vi "Codec_defaultJSON.vi"(8 "error in (no error)":errorcluster, 11 "SecureMqttCodec in":refnum<class "SecureMqttCodec.lvclass">) -> (0 "error out":errorcluster, 3 "SecureMqttCodec out":refnum<class "SecureMqttCodec.lvclass">)   [LabVIEW 2020, in "SecureMqttCodec.lvclass"]
uses:
  SecureMqttCodec.lvclass
  SecureMqttCodec.lvclass/SecureMqttCodec.ctl
  <vilib>/addons/JSON API/JSON Value/Set from JSON string.vi
  <vilib>/LabVIEW Open Source Project/Epoch Date & Time/epoch.UNIX/Epoch.UNIX.lvclass
  C:/Program Files/National Instruments/LabVIEW 2020/vi.lib/LabVIEW Open Source Project/Epoch Date & Time/epoch/Epoch.lvclass
  <vilib>/addons/JSON API/JSON Scalar/JSON Scalar.lvclass
  C:/Program Files/National Instruments/LabVIEW 2020/vi.lib/addons/JSON API/JSON Value/JSON Value.lvclass
  <vilib>/LabVIEW Open Source Project/Epoch Date & Time/Get Epoch Time.vi
  <vilib>/addons/JSON API/JSON Scalar/Set I64.vi
  <vilib>/addons/JSON API/JSON Scalar/Set String.vi
  <vilib>/addons/JSON API/JSON Value/JSON Value.lvclass
  <vilib>/addons/JSON API/Get Polymorphic/JSON GetSet.lvlib
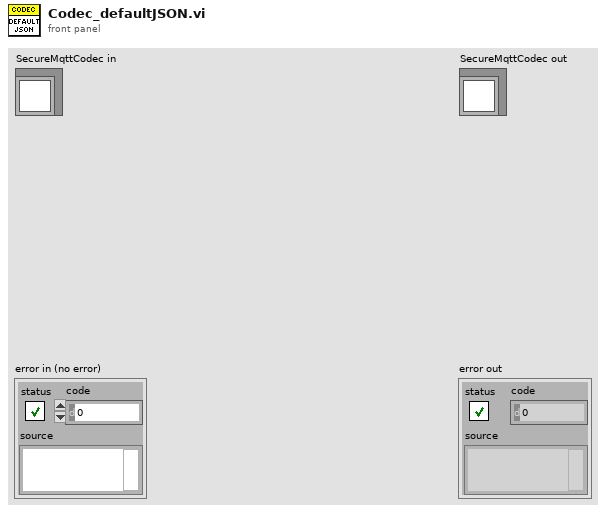
[diagram p1: front panel]
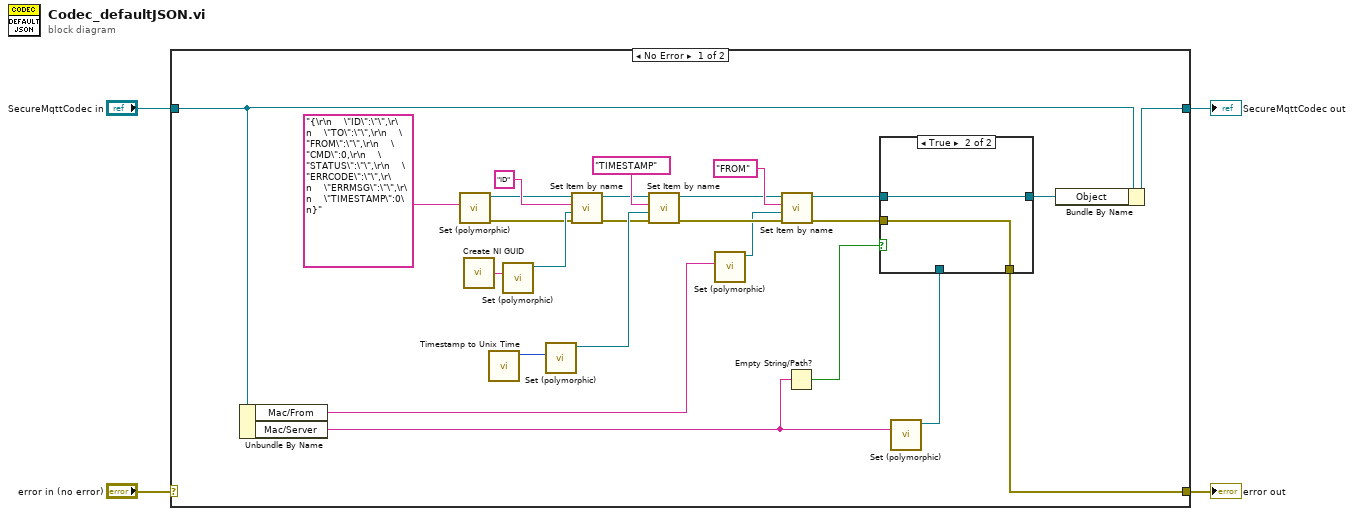
[diagram p0: block diagram]
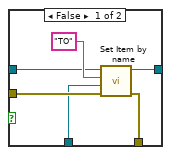
[diagram p2: hidden frame]
diagram:
  n1 = case shown="No Error" "error in (no error)" {
    selector: "error in (no error)" -> [_ w39]
    tunnel: [w27 w39] -> w3
    tunnel: [w28 w38] -> w1
    tunnel: "SecureMqttCodec in" -> [w29 w38]
    frame No Error {
      n2 = Unbundle By Name(w29) -> ("Mac/From"=w9:string, "Mac/Server"=w6:string)
      n3 = call-poly <vilib>:"Set (polymorphic).vi"("JSON stream"="{\r\n    \"ID\":\"\",\r\n    \"TO\":\"\",\r\n    \"FROM\":\"\",\r\n    \"CMD\":0,\r\n    \"STATUS\":\"\",\r\n    \"ERRCODE\":\"\",\r\n    \"ERRMSG\":\"\",\r\n    \"TIMESTAMP\":0\n}" ("JSON String")) -> ("error out"=w20:errorcluster, "JSON Value out"=w21:refnum<class "JSON Value.lvclass">)  [unwired: 8 in, 1 out]
      n4 = call <vilib>:"Create NI GUID.vi"() -> ("NI GUID"=w24:string)
      n5 = call <vilib>:"Timestamp to Unix Time.vi"() -> ("Unix Time (s)"=w19:i64)  [unwired: 10 in, 1 out]
      n6 = call-poly <vilib>:"Set (polymorphic).vi"("String"=w24) -> ("JSON Scalar out"=w23:refnum<class "JSON Scalar.lvclass">)  [unwired: 9 in, 1 out]
      n7 = call-poly <vilib>:"Set (polymorphic).vi"("Numeric"=w19) -> ("JSON Scalar out"=w18:refnum<class "JSON Scalar.lvclass">)  [unwired: 9 in, 1 out]
      n8 = call-dynamic "Set Item by name.vi"("error in (no error)"=w20, "Value"=w23, "name"="ID", "JSON Value In"=w21) -> ("error out"=w15:errorcluster, "JSON Value Out"=w16:refnum<class "JSON Value.lvclass">)  [unwired: 5 in, 1 out]
      n9 = call-dynamic "Set Item by name.vi"("error in (no error)"=w15, "Value"=w18, "name"="TIMESTAMP", "JSON Value In"=w16) -> ("error out"=w10:errorcluster, "JSON Value Out"=w13:refnum<class "JSON Value.lvclass">)  [unwired: 5 in, 1 out]
      n10 = call-poly <vilib>:"Set (polymorphic).vi"("String"=w9) -> ("JSON Scalar out"=w8:refnum<class "JSON Scalar.lvclass">)  [unwired: 9 in, 1 out]
      n11 = call-dynamic "Set Item by name.vi"("error in (no error)"=w10, "Value"=w8, "name"="FROM", "JSON Value In"=w13) -> ("error out"=w11:errorcluster, "JSON Value Out"=w12:refnum<class "JSON Value.lvclass">)  [unwired: 5 in, 1 out]
      n12 = Empty String/Path?(string/path=w6) -> (empty?=w5:bool)
      n13 = call-poly <vilib>:"Set (polymorphic).vi"("String"=w6) -> ("JSON Scalar out"=w7:refnum<class "JSON Scalar.lvclass">)  [unwired: 9 in, 1 out]
      n14 = case shown="True" w5 {
        tunnel: [w35 w36] -> w27
        tunnel: [w34 w37] -> w26
        tunnel: w12 -> [w32 w37]
        tunnel: w11 -> [w31 w36]
        tunnel: w7 -> [w30 _]
        frame False {
          n15 = call-dynamic "Set Item by name.vi"("error in (no error)"=w31, "Value"=w30, "name"="TO", "JSON Value In"=w32) -> ("error out"=w35:errorcluster, "JSON Value Out"=w34:refnum<class "JSON Value.lvclass">)  [unwired: 5 in, 1 out]
        }
        frame True {
        }
      }
      n16 = Bundle By Name(cluster=w29, "Object"=w26) -> (w28:refnum<class "SecureMqttCodec.lvclass">)
    }
    frame Error {
    }
  }
  "error out" <- w3
  "SecureMqttCodec out" <- w1
